vi "GetCaseRefnum__slk_mt.vi"(8 "error in (no error)":errorcluster, 11 "vi refnum in":refnum<vi>) -> (0 "error out":errorcluster, 2 "not found?":bool, 3 "case refnum out":refnum<vi>)   [LabVIEW 2020, in "Lazyboots Menu Tool.lvlib"]
doc: "Returns case refnum from block diagram selection list of a VI."
uses:
  Library/Lazyboots Menu Tool.lvlib
panel:
  # "GetCaseRefnum__slk_mt.vi\nReturns case refnum from block diagram selection list of a VI.\n\nNOTICE -- YOU MUST LEAVE THIS NOTICE IN PLACE.\n\nCopyright (c) 2011, LIANG LIU Shawn.Liu.cn@gmail.com\nAll rights reserved.\n\nRedistribution and use in source and binary forms, with or without modification, are permitted provided that the following conditions are met:\n-Redistributions of source code must retain the above copyright notice, this list of conditions and the following disclaimer.\n-Redistributions in binary form must reproduce the above copyright notice, this list of conditions and the following disclaimer in the documentation and/or other materials provided with the distribution.\n-Neither the name of the eLp nor the names of its contributors may be used to endorse or promote products derived from this software without specific prior written permission.\n\nTHIS SOFTWARE IS PROVIDED BY THE COPYRIGHT HOLDERS AND CONTRIBUTORS \"AS IS\" AND ANY EXPRESS OR IMPLIED WARRANTIES, INCLUDING, BUT NOT LIMITED TO, THE IMPLIED WARRANTIES OF MERCHANTABILITY AND FITNESS FOR A PARTICULAR PURPOSE ARE DISCLAIMED. IN NO EVENT SHALL THE COPYRIGHT HOLDER OR CONTRIBUTORS BE LIABLE FOR ANY DIRECT, INDIRECT, INCIDENTAL, SPECIAL, EXEMPLARY, OR CONSEQUENTIAL DAMAGES (INCLUDING, BUT NOT LIMITED TO, PROCUREMENT OF SUBSTITUTE GOODS OR SERVICES; LOSS OF USE, DATA, OR PROFITS; OR BUSINESS INTERRUPTION) HOWEVER CAUSED AND ON ANY THEORY OF LIABILITY, WHETHER IN CONTRACT, STRICT LIABILITY, OR TORT (INCLUDING NEGLIGENCE OR OTHERWISE) ARISING IN ANY WAY OUT OF THE USE OF THIS SOFTWARE, EVEN IF ADVISED OF THE POSSIBILITY OF SUCH DAMAGE."
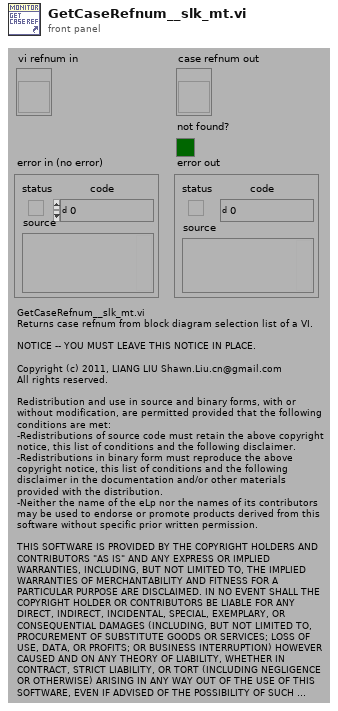
[diagram p1: front panel]
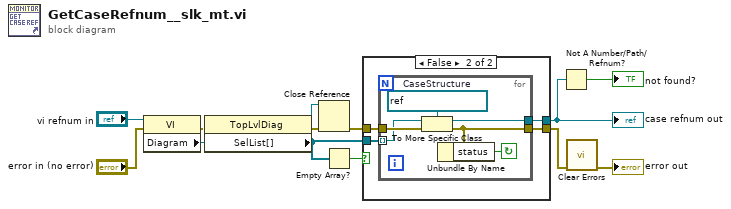
[diagram p0: block diagram]
diagram:
  n1 = property on="Property Node" class="VI"(reference="vi refnum in", error in="error in (no error)") -> (error out=w11:errorcluster, "Diagram"=w13:refnum<vi>)  [unwired: 1 out]
  n2 = property on="Property Node" class="TopLvlDiag"(reference=w13, error in=w11) -> (reference out=w6:refnum<vi>, error out=w12:errorcluster, "SelList[]"=w9:refnum<vi>[])
  n3 = Close Reference(reference=w6, error in (no error)=w12) -> (error out=w7:errorcluster)
  n4 = Empty Array?(array=w9) -> (empty?=w8:bool)
  n5 = case shown="False" w8 {
    tunnel: w9 -> [_ w18]
    tunnel: w7 -> [w14 w17]
    tunnel: [w14 w16] -> w3
    tunnel: [_ w15] -> w5
    frame True {
    }
    frame False {
      n6 = for {
        tunnel: w18 -> [w19] mode=indexing
        tunnel: w17 -> [w23]
        tunnel: [w22] -> w16
        tunnel: [w20] -> w15
        stop <- w21 continue-if-true
        w24 = refnum<vi> refnum  # CaseStructure
        n7 = To More Specific Class(target class=w24, reference=w19, error in=w23) -> (specific class reference=w20:refnum<vi>, error out=w22:errorcluster)
        n8 = Unbundle By Name(w22) -> ("status"=w21:bool)
      }
    }
  }
  "case refnum out" <- w5
  n9 = Not A Number/Path/Refnum?(number/path/refnum=w5) -> (NaN/Path/Refnum?=→"not found?":bool)
  n10 = call <vilib>:"Clear Errors.vi"("error in (no error)"=w3) -> ("error out"=→"error out":errorcluster)  [unwired: 5 in, 1 out]
